vi "Clear.vi"(8 "error in (no error)":errorcluster, 11 "Mock Filter in":refnum<class "Mock Filter.lvclass">) -> (0 "error out":errorcluster, 3 "Mock Filter out":refnum<class "Mock Filter.lvclass">)   [LabVIEW 2020, in "Mock Filter.lvclass"]
uses:
  Mock Filter.lvclass
  Mock Filter.lvclass/Mock Filter.ctl
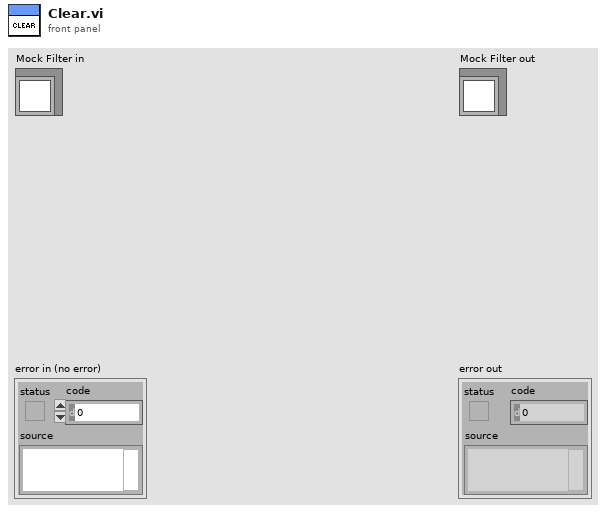
[diagram p1: front panel]
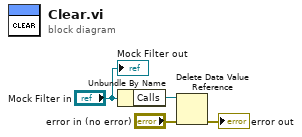
[diagram p0: block diagram]
diagram:
  n1 = Unbundle By Name("Mock Filter in") -> ("Calls"=w3:refnum<data-value>)
  n2 = Delete Data Value Reference(data value reference=w3, error in="error in (no error)") -> (error out=→"error out":errorcluster)  [unwired: 1 out]
  "Mock Filter out" <- "Mock Filter in"
